vi "探头窗口-2-服务器版.vi"() -> ()   [LabVIEW 2013]
panel:
  in  "外部停止命令？":bool=TRUE
  out "引用-监测模式？":refnum<vi>
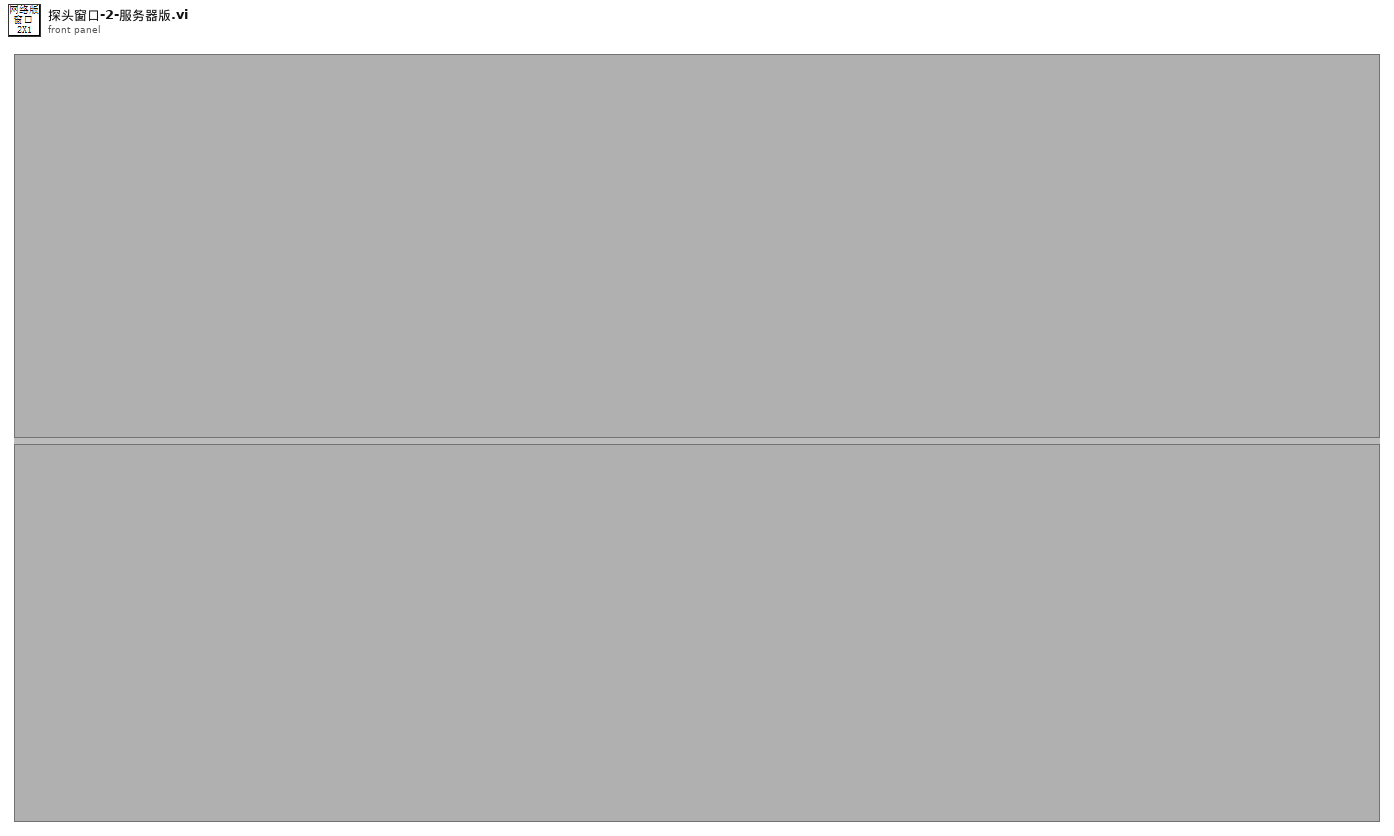
[diagram p1: front panel]
types:
  T1 = enum32{"Invalid", "Standard", "Closed", "Hidden", "Minimized", "Maximized"}
  T2 = cluster{"探头地址与信息":cluster{"网络地址":cluster{"IP":string, "port":u16}, "探头信息":string}, "测量值":cluster{"时间":timestamp, "数值":dbl}, "限值":cluster{"限值1":dbl, "限值2":dbl}, "探头状态":enum16{"正常", "离线", "禁用", "一级报警", "二级报警"}}[]
  T3 = typedef "eventvkey.ctl" = enum16{"ASCII", "Enter", "Return", "Shift", "Ctrl", "Alt", "Cmd", "Opt", "Caps", "NumLock", "Clear", "Break", "Up", "Down", "Left", "Right", "Insert", "Delete", "Home", "End", "PageUp", "PageDown", "Escape", "Help", "Pause", "ScrollLock", "F1", "F2", "F3", "F4", "F5", "F6", "F7", "F8", "F9", "F10", "F11", "F12", "F13", "F14", "F15", "F16", "F17", "F18", "F19", "F20", "F21", "F22", "F23", "F24", "Play", "VolumeUp", "VolumeDown", "Mute", "Two Byte Char"}
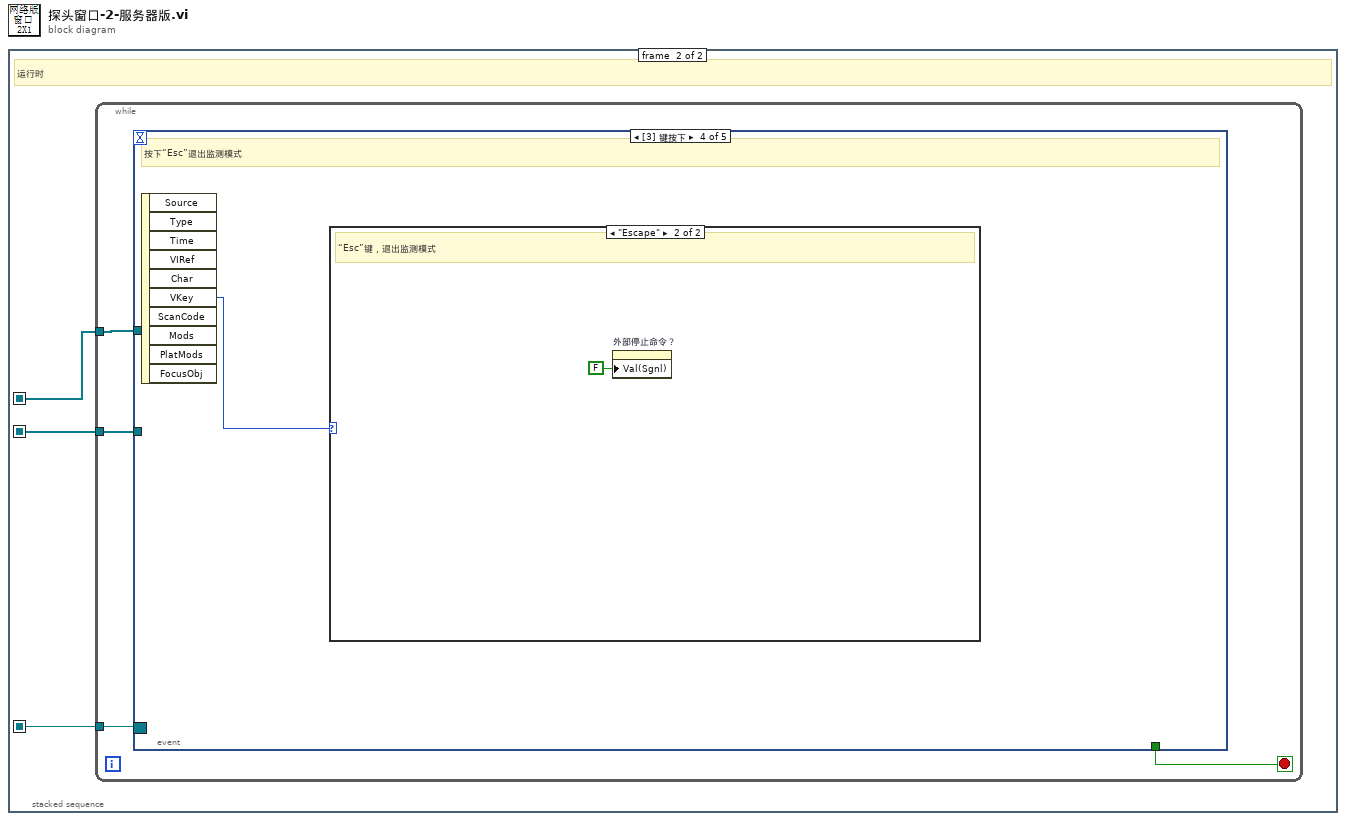
[diagram p0: block diagram]
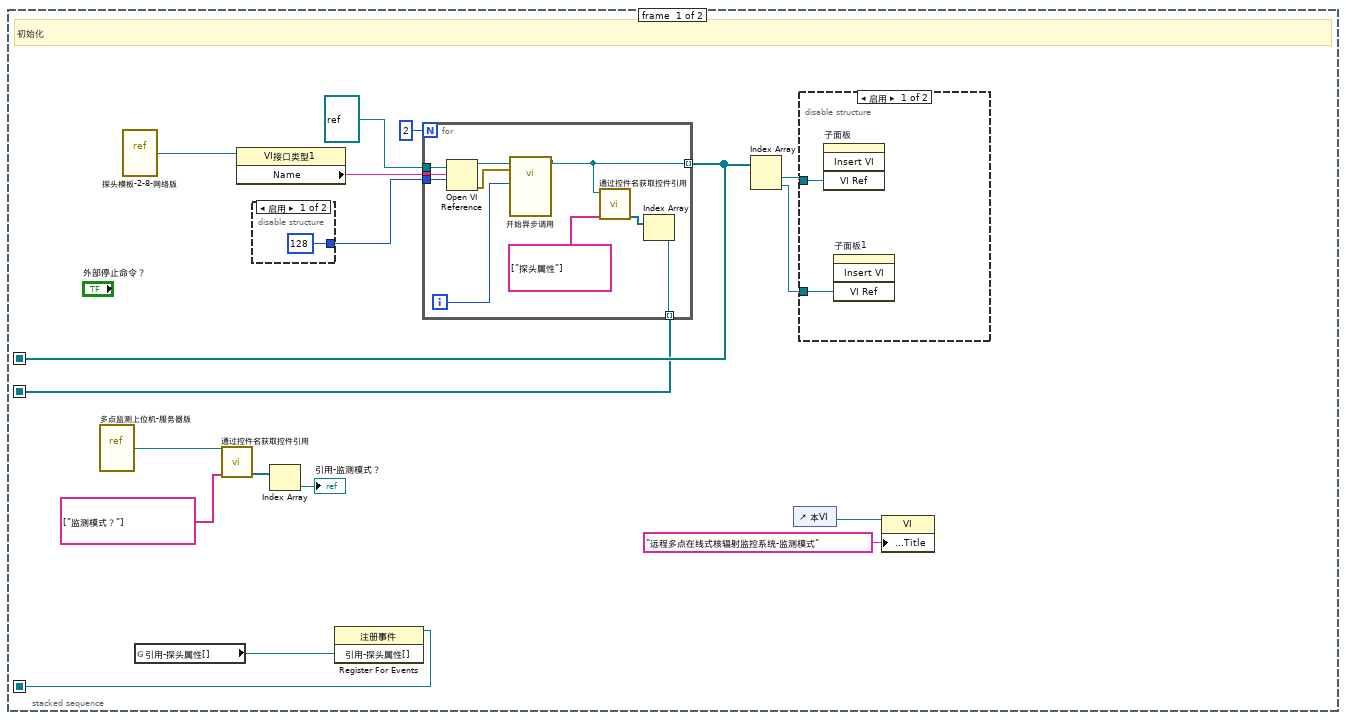
[diagram p2: hidden frame]
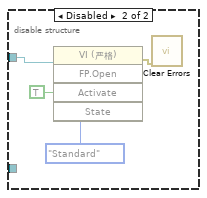
[diagram p3: hidden frame]
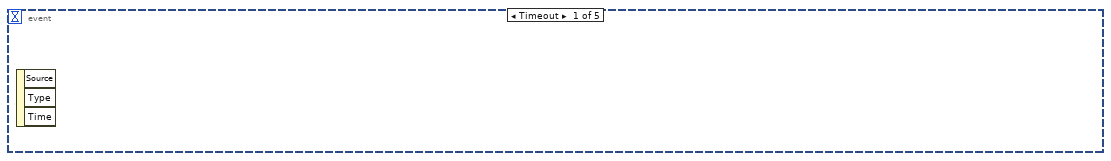
[diagram p5: hidden frame]
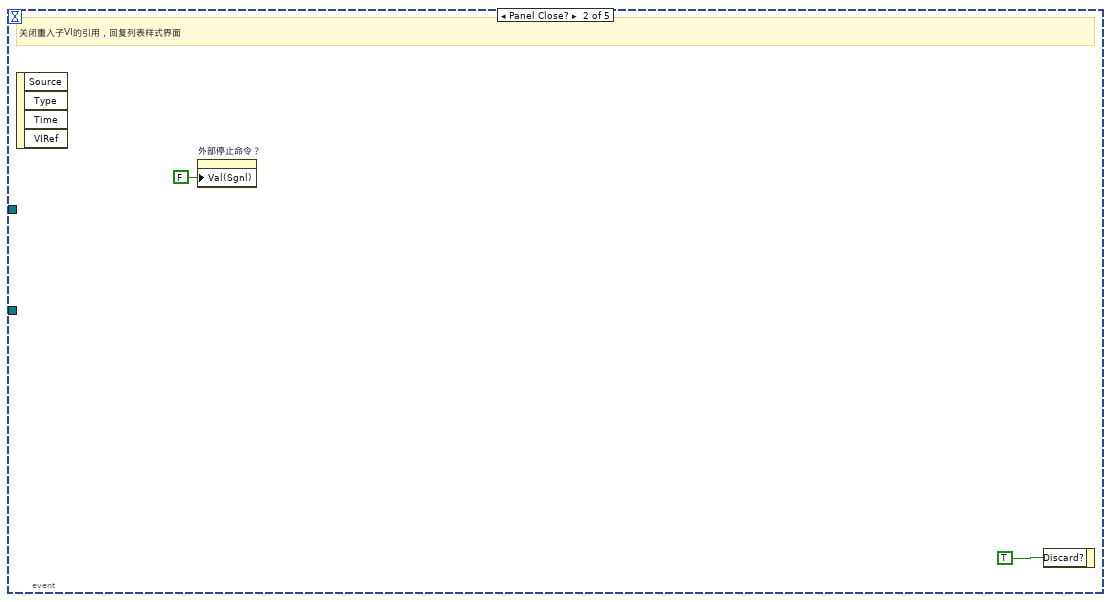
[diagram p6: hidden frame]
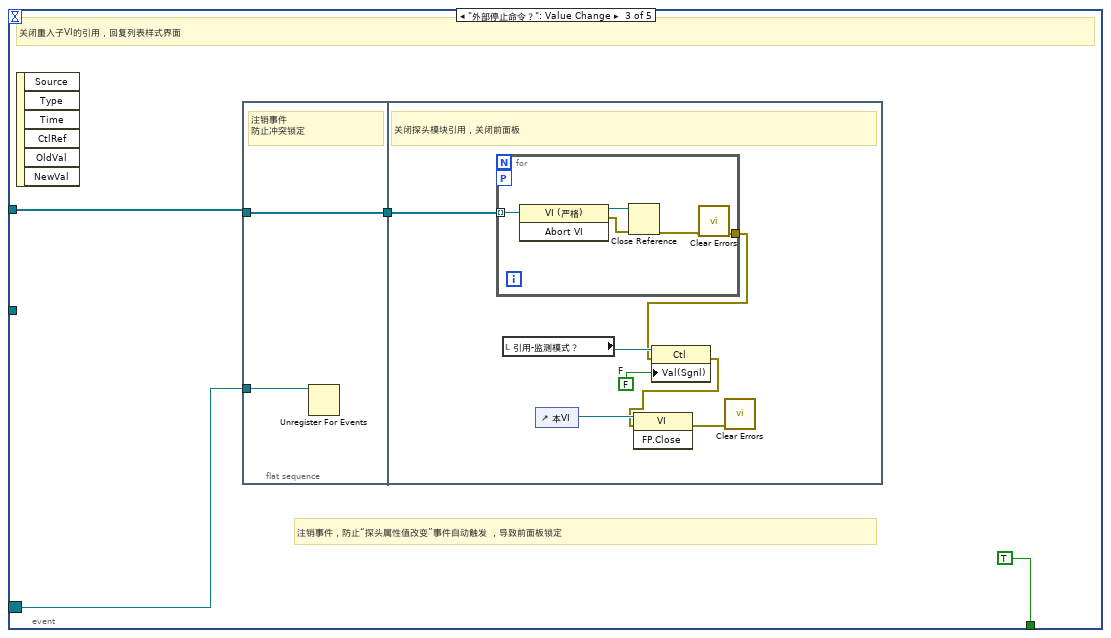
[diagram p7: hidden frame]
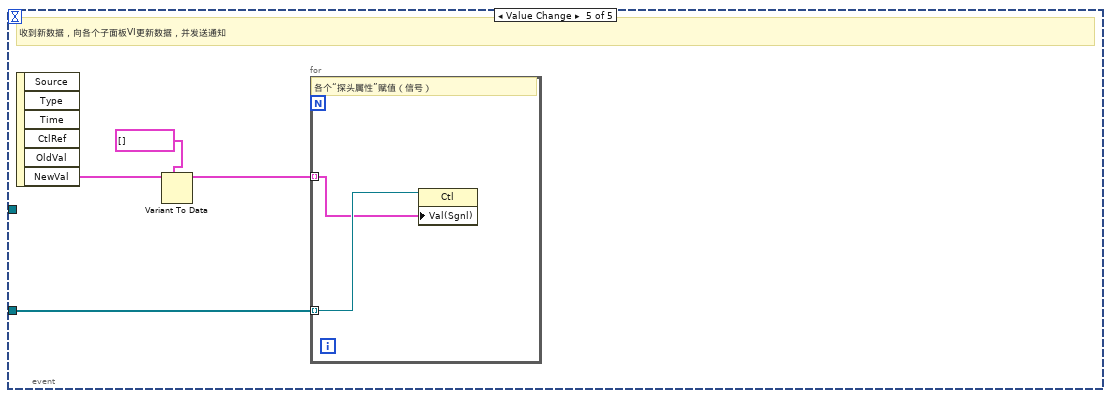
[diagram p9: hidden frame]
diagram:
  n1 = stacked-sequence {
    seq-local: [w14 _] -> [_ w37]
    seq-local: [w6 _] -> [_ w36]
    seq-local: [w4 _] -> [_ w35]
    frame #0 {
      # "初始化"
      n2 = vi-ref "多点监测上位机-服务器版.vi"() -> (w10:refnum<vi>)
      n3 = vi-ref "探头模板-2-8-网络版.vi"() -> (w17:refnum<vi>)
      n4 = global read "全局变量-35点监测.vi" "引用-探头属性[]"() -> (w3:refnum<vi>)
      n5 = call "通过控件名获取控件引用.vi"("控件名数组"=string[] ["监测模式？"], "VI引用"=w10) -> ("控件引用输出"=w8:refnum<vi>[])  [unwired: 7 in, 2 out]
      n6 = property class="VI接口类型1"(reference=w17) -> ("Name"=w16:string)  [unwired: 1 in, 2 out]
      n7 = disable-structure shown="启用" {
        disable-tunnel: [128 ("选项") _] -> w15
        frame Enabled {
        }
        frame Disabled {
        }
      }
      n8 = Index Array(array=w8) -> (element=→"引用-监测模式？":refnum<vi>)  [unwired: 1 in]
      n9 = register-events(w3) -> (reference out=w4:refnum<event-registration>)  [unwired: 2 in, 1 out]
      n10 = for "For循环" {
        N: 2 -> [_]
        tunnel: w16 -> [w34]
        tunnel: w15 -> [w33]
        tunnel: refnum<vi> refnum ("类型说明符VI引用句柄（仅用于类型）") -> [w32]
        tunnel: [w27] -> w14 mode=indexing
        tunnel: [w29] -> w6 mode=indexing
        i -> [w26]
        n11 = Open VI Reference(type specifier VI Refnum (for type only)=w32, vi path=w34, options=w33) -> (vi reference=w28:refnum<vi>, error out=w25:errorcluster)  [unwired: 3 in]
        n12 = call-by-ref "开始异步调用"(reference=w28, error in=w25, "探头序号"=w26) -> (reference out=w27:refnum<vi>)  [unwired: 11 in, 1 out]
        n13 = call "通过控件名获取控件引用.vi"("控件名数组"=string[] ["探头属性"], "VI引用"=w27) -> ("控件引用输出"=w30:refnum<vi>[])  [unwired: 7 in, 2 out]
        n14 = Index Array(array=w30) -> (element=w29:refnum<vi>)  [unwired: 1 in]
      }
      n15 = Index Array(array=w14) -> (element #1=w13:refnum<vi>, element #2=w12:refnum<vi>)  [unwired: 2 in]
      n16 = control-ref of="本VI"() -> (w2:refnum<vi>)
      n17 = disable-structure shown="启用" {
        disable-tunnel: w13 -> [w19 w23]
        disable-tunnel: w12 -> [w18 _]
        frame Enabled {
          n18 = invoke on="子面板" class="子面板" method="Insert VI"("VI Ref"=w19) -> ()  [unwired: 3 in, 4 out]
          n19 = invoke on="子面板1" class="SubPnl" method="Insert VI"("VI Ref"=w18) -> ()  [unwired: 3 in, 4 out]
        }
        frame Disabled {
          n20 = invoke class="VI (严格)" method="FP.Open"(reference=w23, "Activate"=TRUE ("激活？"), "State"=T1."Standard" ("状态")) -> (error out=w20:errorcluster)  [unwired: 2 in, 4 out]
          n21 = call <vilib>:"Clear Errors.vi"("error in (no error)"=w20) -> ()  [unwired: 6 in, 1 out]
        }
      }
      n22 = property class="VI"(reference=w2, "Front Panel.Title"="远程多点在线式核辐射监控系统-监测模式" ("前面板窗口:标题")) -> ()  [unwired: 1 in, 2 out]
    }
    frame #1 {
      # "运行时"
      n23 = while {
        tunnel: w37 -> [w40]
        tunnel: w36 -> [w39]
        tunnel: w35 -> [w38]
        stop <- w41 stop-if-true
        n24 = event shown="[3] 键按下" {
          selector: w38 -> [_ _ w44 _ _]
          dyn-events: _ -> [_ _ _ _ _]
          timeout: _ -> [_ _ _ _ _]
          tunnel: [_ _ TRUE ("放弃？") _ _] -> w41
          tunnel: w40 -> [_ _ w46 _ _]
          tunnel: w39 -> [_ _ _ _ w67]
          event Timeout {
            n25 = event-data() -> ()  [unwired: 1 in, 3 out]
          }
          event Panel Close? {
            # "关闭重入子VI的引用，回复列表样式界面"
            n26 = event-data() -> ()  [unwired: 1 in, 4 out]
            n27 = property on="外部停止命令？" class="Bool (严格)"("Val(Sgnl)"=FALSE ("值(信号)")) -> ()  [unwired: 2 in, 2 out]
            n28 = event-data("Discard?"=TRUE ("放弃？")) -> ()  [unwired: 1 in, 1 out]
          }
          event "外部停止命令？": Value Change {
            # "注销事件，防止“探头属性值改变”事件自动触发 ，导致前面板锁定"
            # "关闭重入子VI的引用，回复列表样式界面"
            n29 = event-data() -> ()  [unwired: 1 in, 6 out]
            n30 = flat-sequence {
              tunnel: w46 -> [w49]
              tunnel: [w49] -> w45
              tunnel: w44 -> [w48]
              tunnel: w45 -> [w56]
              frame #0 {
                # "注销事件\n防止冲突锁定"
                n31 = Unregister For Events(event registration refnum=w48) -> ()  [unwired: 1 in, 1 out]
              }
              frame #1 {
                w54 = FALSE  # F
                # "关闭探头模块引用，关闭前面板"
                n32 = for "For循环" {
                  tunnel: w56 -> [w61] mode=indexing
                  workers-P: _ -> [_]
                  tunnel: [w57] -> w52
                  n33 = invoke class="VI (严格)" method="Abort VI"(reference=w61) -> (reference out=w60:refnum<vi>, error out=w59:errorcluster)  [unwired: 2 in, 1 out]
                  n34 = Close Reference(reference=w60, error in (no error)=w59) -> (error out=w58:errorcluster)
                  n35 = call <vilib>:"Clear Errors.vi"("error in (no error)"=w58) -> ("error out"=w57:errorcluster)  [unwired: 6 in]
                }
                n36 = local read "引用-监测模式？"() -> (w55:refnum<vi>)
                n37 = control-ref of="本VI"() -> (w53:refnum<vi>)
                n38 = property class="Ctl"(reference=w55, error in=w52, "Val(Sgnl)"=w54) -> (error out=w51:errorcluster)  [unwired: 1 out]
                n39 = invoke class="VI" method="FP.Close"(reference=w53, error in=w51) -> (error out=w50:errorcluster)  [unwired: 1 in, 2 out]
                n40 = call <vilib>:"Clear Errors.vi"("error in (no error)"=w50) -> ()  [unwired: 6 in, 1 out]
              }
            }
          }
          event Key Down {
            # "按下“Esc”退出监测模式"
            n41 = event-data() -> ("VKey"=w62:T3)  [unwired: 1 in, 9 out]
            n42 = case shown="\"Escape\"" w62 {
              frame "ASCII", Default {
              }
              frame "Escape" {
                # "“Esc”键，退出监测模式"
                n43 = property on="外部停止命令？" class="Bool (严格)"("Val(Sgnl)"=FALSE ("值(信号)")) -> ()  [unwired: 2 in, 2 out]
              }
            }
          }
          event Value Change {
            # "收到新数据，向各个子面板VI更新数据，并发送通知"
            n44 = event-data() -> ("NewVal"=w66:T2)  [unwired: 1 in, 5 out]
            n45 = Variant To Data(type=T2 [], Variant=w66) -> (data=w65:T2)  [unwired: 1 in, 1 out]
            n46 = for "For循环" {
              tunnel: w67 -> [w69] mode=indexing
              tunnel: w65 -> [w68] mode=indexing
              # "各个“探头属性”赋值（信号）"
              n47 = property class="Ctl"(reference=w69, "Val(Sgnl)"=w68) -> ()  [unwired: 1 in, 2 out]
            }
          }
        }
      }
    }
  }
